vi "Draw weighted arm.vi"(6 "Setpoint":dbl[unit] format="%#.2g", 8 "Arm parameters":T1={"Mass at end"=1.0, "Length "=0.3, "Gear ratio (out/in)"=10.0, "Initial position"=0.0}, 9 "Motor Position":dbl[unit] format="%#.2g", 10 "Shaft Position":dbl[unit] format="%#.2g", 11 "Shaft pixel  position":cluster{"horizontal":i16, "vertical":i16}={"horizontal"=100, "vertical"=80}) -> (2 "Shaft pixel  position out":cluster{"horizontal":i16, "vertical":i16}={"horizontal"=80, "vertical"=80}, 3 "2D Picture":picture)   [LabVIEW 2019]
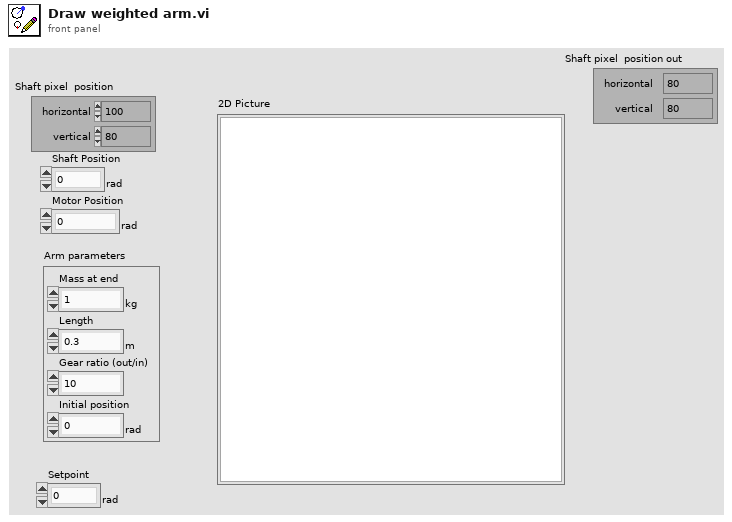
[diagram p1: front panel]
types:
  T1 = cluster{"Mass at end":dbl[unit], "Length ":dbl[unit], "Gear ratio (out/in)":dbl, "Initial position":dbl[unit]}
  T2 = cluster{"Width":u16, "Style":enum32{"Solid", "Dash", "Dot", "DashDot", "DashDotDot"}}
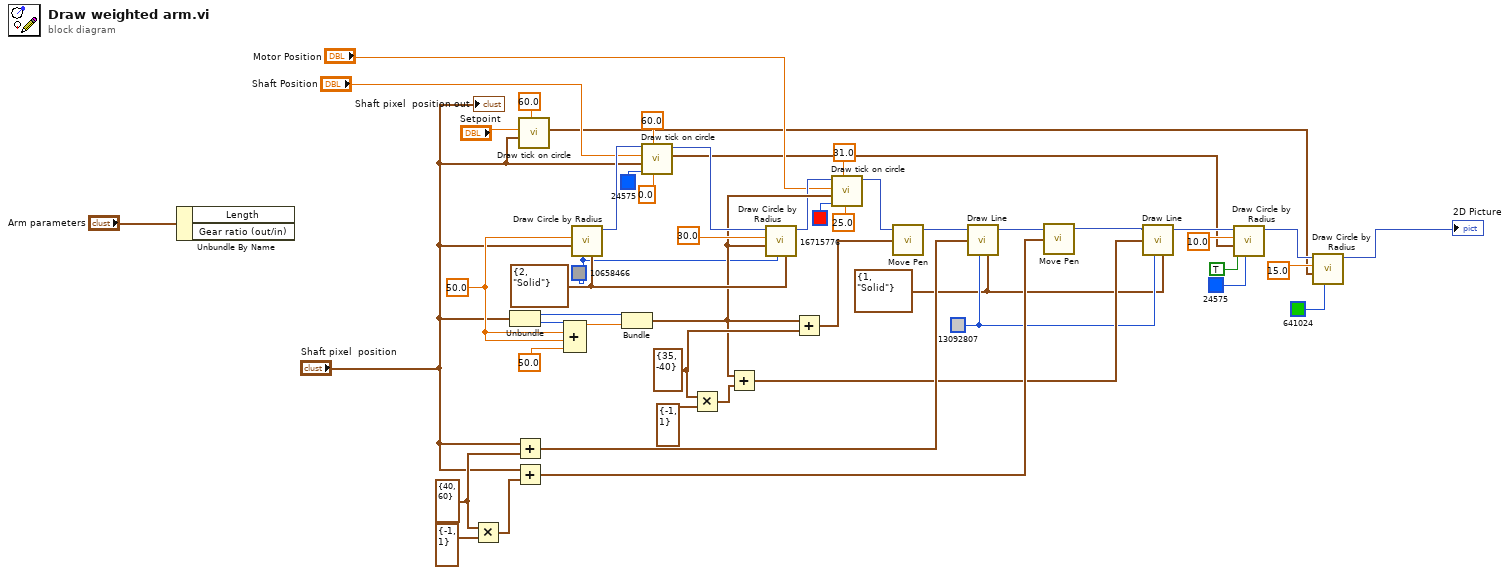
[diagram p0: block diagram]
diagram:
  w10 = u32 10658466 ("color(black)")
  w28 = T2 {"Width"=1, "Style"=enum."Solid"} ("pen")
  w29 = T2 {"Width"=2, "Style"=enum."Solid"} ("pen")
  w30 = u32 13092807
  w33 = cluster{"horizontal":i16, "vertical":i16} {"horizontal"=35, "vertical"=-40} ("y")
  w37 = cluster{"horizontal":i16, "vertical":i16} {"horizontal"=40, "vertical"=60} ("y")
  w45 = 50.0
  n1 = Unbundle By Name("Arm parameters") -> ()  [unwired: 2 out]
  n2 = Multiply(x=w37, y=cluster{"horizontal":i16, "vertical":i16} {"horizontal"=-1, "vertical"=1}) -> (x*y=w36:cluster{"horizontal":i16, "vertical":i16})
  n3 = Unbundle("Shaft pixel  position") -> ("horizontal"=w49:i16, "vertical"=w48:i16)
  n4 = Add(x="Shaft pixel  position", y=w37) -> (x+y=w41:cluster{"horizontal":i16, "vertical":i16})
  n5 = Add(x="Shaft pixel  position", y=w36) -> (x+y=w35:cluster{"horizontal":i16, "vertical":i16})
  n6 = call "Draw tick on circle.vi"("outer radius"=60.0, "Shaft Position"="Shaft pixel  position", "Motor Position"="Setpoint") -> ("outer tick"=w3:cluster{dbl, dbl})  [unwired: 7 in, 1 out]
  n7 = Compound Arithmetic op=unknown(w48, w45, w45, 50.0) -> (w46:dbl)
  n8 = call <vilib>:"Draw Circle by Radius.vi"("pen"=w29, "color(black)"=w10, "pixel center"="Shaft pixel  position", "radius"=w45) -> ("new picture"=w25:picture)  [unwired: 7 in]
  n9 = Bundle("horizontal"=w49, w46) -> (w23:cluster{"horizontal":i16, dbl})  [unwired: 1 in]
  n10 = call "Draw tick on circle.vi"("inner radius"=0.0, "outer radius"=60.0, "color"=u32 24575, "Shaft Position"="Shaft pixel  position", "Motor Position"="Shaft Position", "picture in"=w25) -> ("outer tick"=w2:cluster{dbl, dbl}, "picture out"=w24:picture)  [unwired: 4 in]
  n11 = Multiply(x=w33, y=cluster{"horizontal":i16, "vertical":i16} {"horizontal"=-1, "vertical"=1}) -> (x*y=w32:cluster{"horizontal":i16, "vertical":i16})
  n12 = Add(x=w23, y=w32) -> (x+y=w31:cluster{"horizontal":i16, dbl})
  n13 = call <vilib>:"Draw Circle by Radius.vi"("pen"=w29, "color(black)"=w10, "pixel center"=w23, "radius"=30.0, "picture"=w24) -> ("new picture"=w22:picture)  [unwired: 6 in]
  n14 = Add(x=w23, y=w33) -> (x+y=w42:cluster{"horizontal":i16, dbl})
  n15 = call "Draw tick on circle.vi"("inner radius"=25.0, "outer radius"=31.0, "color"=u32 16715776, "Shaft Position"=w23, "Motor Position"="Motor Position", "picture in"=w22) -> ("picture out"=w21:picture)  [unwired: 4 in, 1 out]
  n16 = call <vilib>:"Move Pen.vi"("new position"=w42, "picture"=w21) -> ("new picture"=w43:picture)  [unwired: 3 in]
  n17 = call <vilib>:"Draw Line.vi"("picture"=w43, "end point"=w41, "color(black)"=w30, "pen"=w28) -> ("new picture"=w40:picture)  [unwired: 5 in]
  n18 = call <vilib>:"Move Pen.vi"("new position"=w35, "picture"=w40) -> ("new picture"=w39:picture)  [unwired: 3 in]
  n19 = call <vilib>:"Draw Line.vi"("picture"=w39, "end point"=w31, "color(black)"=w30, "pen"=w28) -> ("new picture"=w14:picture)  [unwired: 5 in]
  n20 = call <vilib>:"Draw Circle by Radius.vi"("color(black)"=u32 24575, "fill?(F)"=TRUE, "pixel center"=w2, "radius"=10.0, "picture"=w14) -> ("new picture"=w9:picture)  [unwired: 6 in]
  n21 = call <vilib>:"Draw Circle by Radius.vi"("color(black)"=u32 641024, "pixel center"=w3, "radius"=15.0, "picture"=w9) -> ("new picture"=→"2D Picture":picture)  [unwired: 7 in]
  "Shaft pixel  position out" <- "Shaft pixel  position"
